vi "Add active channel values into data array.vi"(8 "Module":i32, 9 "Active channels":T1(array[cluster])=[{"Active channels"=[], "Memory offset"=0}, {"Active channels"=[], "Memory offset"=0}, {"Active channels"=[], "Memory offset"=0}, {"Active channels"=[], "Memory offset"=0}, {"Active channels"=[], "Memory offset"=0}, {"Active channels"=[], "Memory offset"=0}, {"Active channels"=[], "Memory offset"=0}, {"Active channels"=[], "Memory offset"=0}], 10 "Acquired data":sgl[](array[numeric])=[0.0, 0.0, 0.0, 0.0, 0.0, 0.0, 0.0, 0.0, 0.0, 0.0, 0.0, 0.0, 0.0, 0.0, 0.0, 0.0, 0.0, 0.0, 0.0, 0.0, 0.0, 0.0, 0.0, 0.0, 0.0, 0.0, 0.0, 0.0, 0.0, 0.0, 0.0, 0.0], 11 "Memory data":sgl[](array[numeric])=[0.0, 0.0, 0.0, 0.0, 0.0, 0.0, 0.0, 0.0, 0.0, 0.0, 0.0, 0.0, 0.0, 0.0, 0.0, 0.0, 0.0, 0.0, 0.0, 0.0, 0.0, 0.0, 0.0, 0.0, 0.0, 0.0, 0.0, 0.0, 0.0, 0.0, 0.0, 0.0]) -> (3 "Updated data":sgl[](array[numeric]))   [LabVIEW 2018]
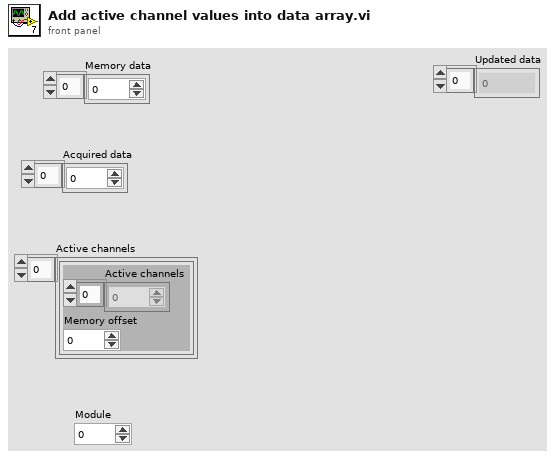
[diagram p1: front panel]
types:
  T1 = cluster{"Active channels":u8[], "Memory offset":i16}[]
  T2 = cluster{"Active channels":u8[], "Memory offset":i16}
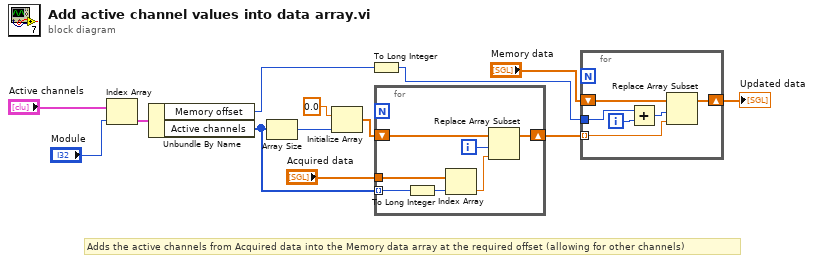
[diagram p0: block diagram]
diagram:
  # "Adds the active channels from Acquired data into the Memory data array at the required offset (allowing for other channels)"
  n1 = Index Array(array="Active channels", index="Module") -> (element=w13:T2)
  n2 = Unbundle By Name(w13) -> ("Memory offset"=w5:i16, "Active channels"=w8:u8[])
  n3 = Array Size(array=w8) -> (size(s)=w11:i32)
  n4 = Initialize Array(sgl 0.0, w11) -> (w9:sgl[])
  n5 = To Long Integer(number=w5) -> (32bit integer=w3:i32)
  n6 = for {
    tunnel: "Acquired data" -> [w20]
    shift-right: [w16] -> w2
    shift-left: w9 -> [w19]
    tunnel: w8 -> [w15] mode=indexing
    i -> [w17]
    n7 = To Long Integer(number=w15) -> (32bit integer=w14:i32)
    n8 = Index Array(array=w20, index=w14) -> (element=w18:sgl)
    n9 = Replace Array Subset(array=w19, new element=w18, index=w17) -> (w16:sgl[])
  }
  n10 = for {
    shift-right: [w25] -> w1
    shift-left: "Memory data" -> [w26]
    tunnel: w3 -> [w24]
    tunnel: w2 -> [w21] mode=indexing
    i -> [w23]
    n11 = Add(x=w24, y=w23) -> (x+y=w22:i32)
    n12 = Replace Array Subset(array=w26, new element=w21, index=w22) -> (w25:sgl[])
  }
  "Updated data" <- w1
